vi "APIReEscribir datos en Google Sheets_boleto.vi"(0 "fila":i32) -> ()   [LabVIEW 2025]
uses:
  <vilib>/httpClient/PUTBuffer.vi
  <vilib>/httpClient/LabVIEWHTTPClient.lvlib
panel:
  out "write_response":string
  out "write_url":string
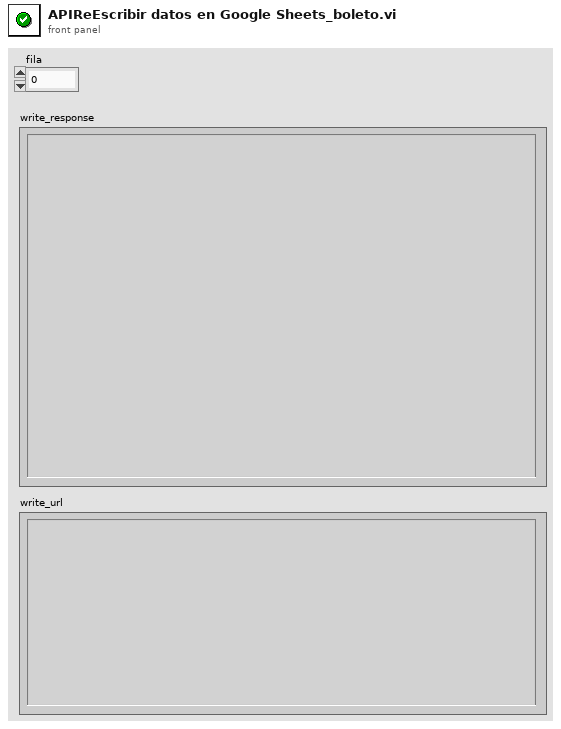
[diagram p1: front panel]
types:
  T1 = typedef "LabVIEWHTTPClient.lvlib/ClientHandle.ctl" = refnum<k1>
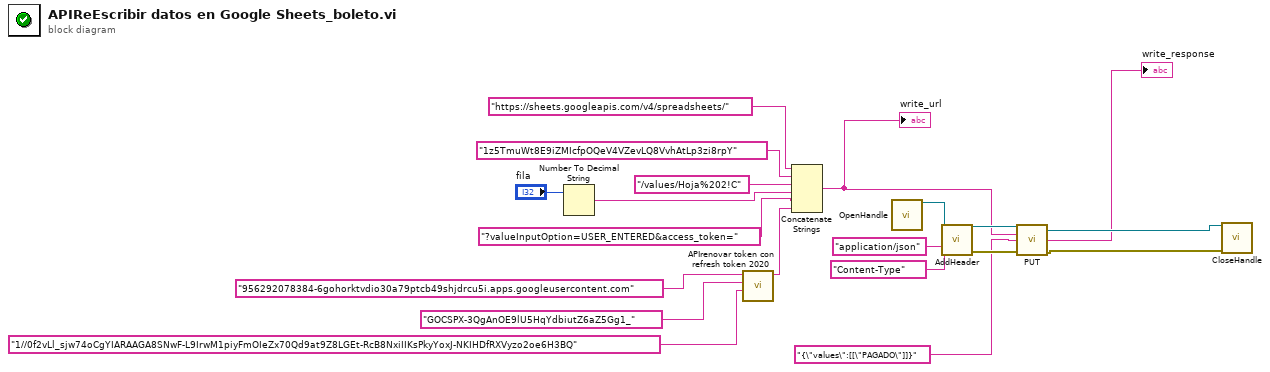
[diagram p0: block diagram]
diagram:
  n1 = Number To Decimal String(number="fila") -> (decimal integer string=w5:string)  [unwired: 1 in]
  n2 = call "APIrenovar token con refresh token 2020.vi"("refresh_token"="1//0f2vLl_sjw74oCgYIARAAGA8SNwF-L9IrwM1piyFmOIeZx70Qd9at9Z8LGEt-RcB8NxiIIKsPkyYoxJ-NKIHDfRXVyzo2oe6H3BQ", "client_secret"="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", "client_id"="956292078384-6gohorktvdio30a79ptcb49shjdrcu5i.apps.googleusercontent.com") -> ("access_token"=w8:string)  [unwired: 8 in]
  n3 = Concatenate Strings("https://sheets.googleapis.com/v4/spreadsheets/", "1z5TmuWt8E9iZMIcfpOQeV4VZevLQ8VvhAtLp3zi8rpY" ("spreadsheet_id"), "/values/Hoja%202!C", w5, "?valueInputOption=USER_ENTERED&access_token=", w8) -> (w10:string)
  "write_url" <- w10
  n4 = call <vilib>:"OpenHandle.vi"() -> ("client handle out"=w17:T1)  [unwired: 14 in, 1 out]
  n5 = call <vilib>:"AddHeader.vi"("client handle"=w17, "header"="Content-Type", "value"="application/json") -> ("client handle out"=w14:T1, "error out"=w13:errorcluster)  [unwired: 11 in]
  n6 = call-poly <vilib>:"PUT.vi"("client handle"=w14, "url"=w10, "buffer"="{\"values\":[[\"PAGADO\"]]}" ("format string"), "error in (no error)"=w13) -> ("client handle out"=w12:T1, "body"=→"write_response":string, "error out"=w11:errorcluster)  [unwired: 8 in, 1 out]
  n7 = call <vilib>:"CloseHandle.vi"("client handle"=w12, "error in (no error)"=w11) -> ()  [unwired: 13 in, 1 out]
